vi "Measurement Logic.vi"() -> ()   [LabVIEW 2021, in "Crosstalk_PMIC.lvlib"]
uses:
  Crosstalk_PMIC.lvlib
  Measurement Configuration.ctl
  Measurement Results.ctl
  <vilib>/MeasurementLink/MeasurementLink Measurement Server/Measure Call Context/Measure Call Context.lvclass
  <instrlib>/niDCPower/nidcpower.llb/niDCPower Sense.ctl
  <instrlib>/niDCPower/nidcpower.llb/niDCPower Source Mode.ctl
  <instrlib>/niDCPower/nidcpower.llb/niDCPower Wait For Event - Event.ctl
  <instrlib>/niDCPower/nidcpower.llb/niDCPower Measurement Type.ctl
  <instrlib>/niScope/Controls/niScope vertical coupling.ctl
  <instrlib>/niScope/Controls/niScope trigger slope.ctl
  <instrlib>/niScope/Controls/niScope trigger coupling.ctl
  <instrlib>/niScope/Controls/niScope trigger source.ctl
  <instrlib>/niDCPower/nidcpower.llb/niDCPower Get Channel Name From String.vi
  <instrlib>/niScope/Configure/Trigger/niScope Configure Trigger Edge.vi
  <instrlib>/niScope/Acquire/Fetch/niScope Multi Fetch WDT.vi
  <vilib>/MeasurementLink/MeasurementLink Measurement Server/Measure Call Context/Accessor/Is Canceled.vi
panel:
  out "CrosstalkGraph":waveform(dbl)[](graph) caption="Ripple"
  out "measure call context out":refnum<class "Measure Call Context.lvclass">
  in  "measure call context in":refnum<class "Measure Call Context.lvclass">
  out "measurement results":T1
  in  "measurement configuration":T2={"Mode of operation"=enum."Perform measurement", "DUT setup time"=1.0, "Aperture time"=0.005, "Source resource name"="", "Source voltage level"=6.0, "Source current limit"=25.0, "Load resource name"="", "Load voltage limit range"=6.0, "Load current level"=0.005, "Scope resource names"=[], "Scope channel names"=[], "Scope sample rate"=10000.0, "Scope acquisition time"=3.0, "Scope probe attenuation"=1.0, "ExportData"=FALSE}
  out "error out":errorcluster
  in  "error in":errorcluster
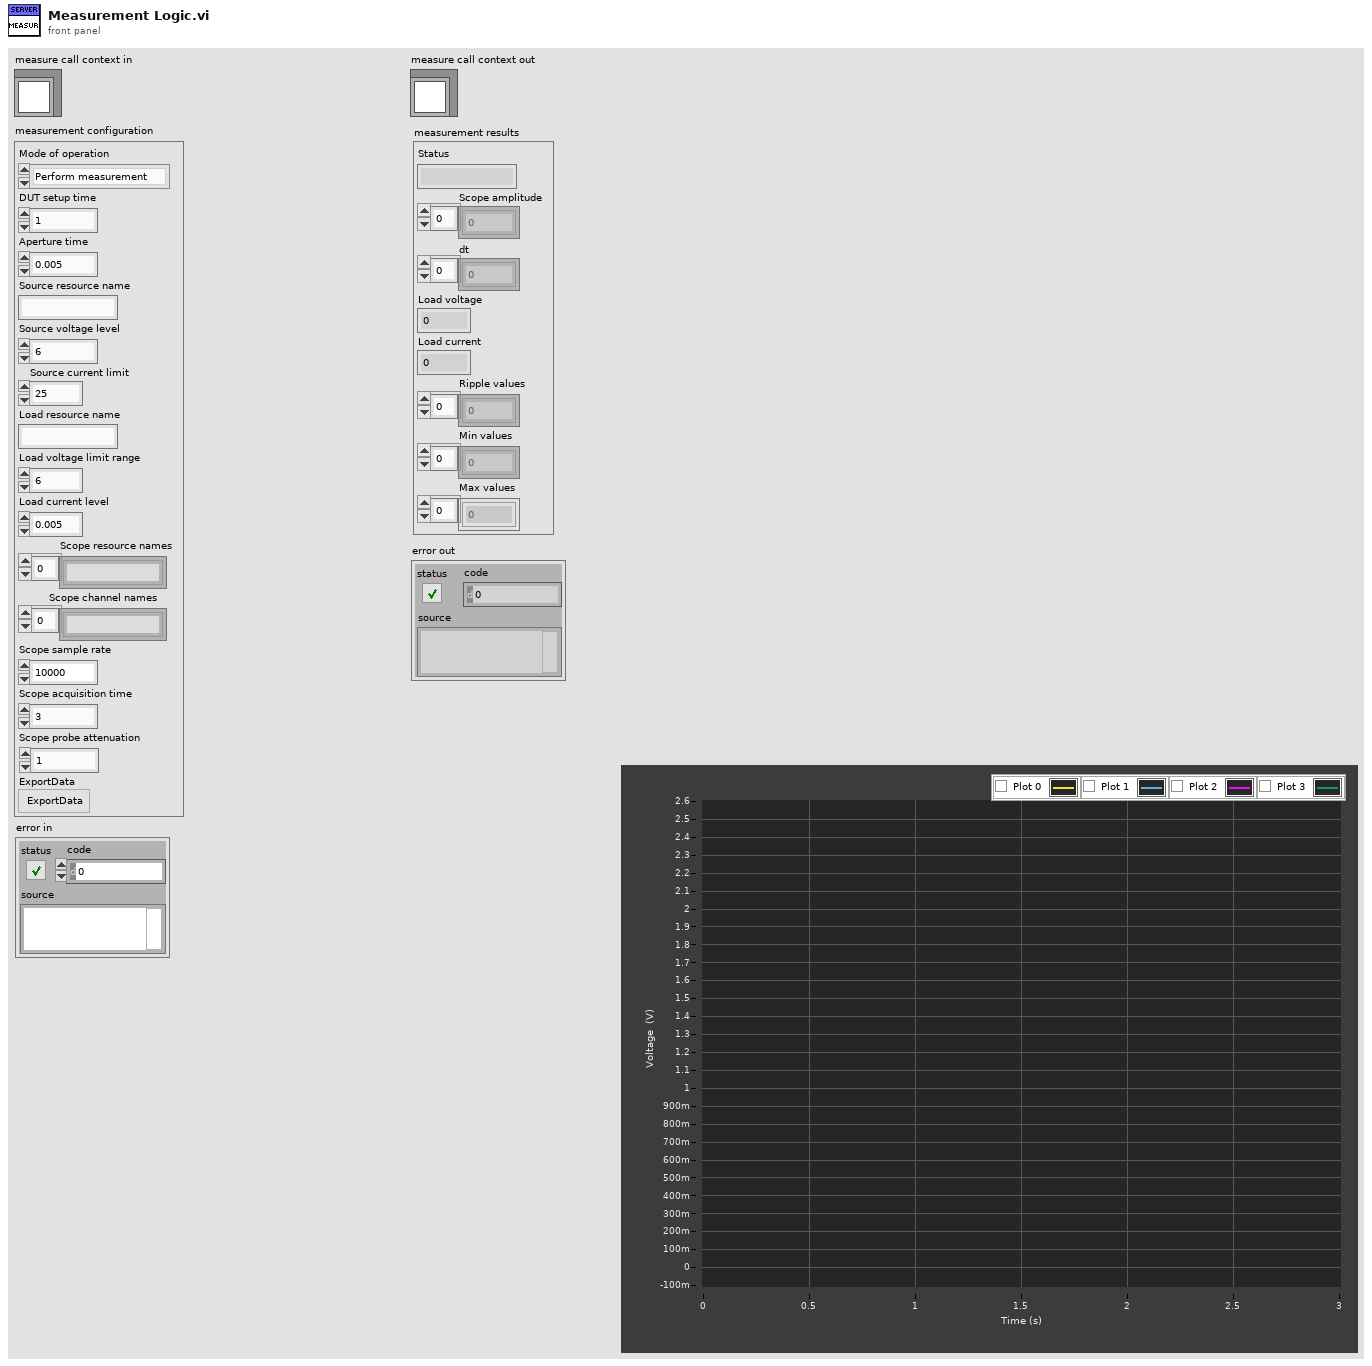
[diagram p1: front panel]
types:
  T1 = typedef "Crosstalk_PMIC.lvlib/Measurement Results.ctl" = cluster{"Status":string, "Scope amplitude":dbl[], "dt":dbl[], "Load voltage":dbl, "Load current":dbl, "Ripple values":dbl[], "Min values":dbl[], "Max values":dbl[]}
  T2 = typedef "Crosstalk_PMIC.lvlib/Measurement Configuration.ctl" = cluster{"Mode of operation":enum32{"Power on the DUT", "Perform measurement", "Power off the DUT"}, "DUT setup time":dbl, "Aperture time":dbl, "Source resource name":string, "Source voltage level":dbl, "Source current limit":dbl, "Load resource name":string, "Load voltage limit range":dbl, "Load current level":dbl, "Scope resource names":string[], "Scope channel names":string[], "Scope sample rate":dbl, "Scope acquisition time":dbl, "Scope probe attenuation":dbl, "ExportData":bool}
  T3 = cluster{"Source out":refnum<k15>, "Source channel name":string, "Load out":refnum<k15>, "Load channel name":string, "Scopes out":refnum<k15>[], "Scope channel names":string[], "Measurement Results":T1}
  T4 = enum32{"Power on the DUT", "Perform measurement", "Power off the DUT"}
  T5 = typedef "niScope trigger source.ctl" = string
  T6 = enum16{"open", "replace", "create", "open or create", "replace or create", "replace or create with confirmation"}
  T7 = typedef "niDCPower Wait For Event - Event.ctl" = i32
  T8 = typedef "niDCPower Source Mode.ctl" = i32
  T9 = typedef "niDCPower Sense.ctl" = i32
  T10 = typedef "niDCPower Measurement Type.ctl" = i32
  T11 = typedef "niScope vertical coupling.ctl" = i32
  T12 = typedef "niScope trigger coupling.ctl" = u16
  T13 = typedef "niScope trigger slope.ctl" = i32
  T14 = typedef "imagedata.ctl" = cluster{"image type":i32, "image depth":i32, "image":u8[], "mask":u8[], "colors":u32[], "Rectangle":cluster{"left":i16, "top":i16, "right":i16, "bottom":i16}}
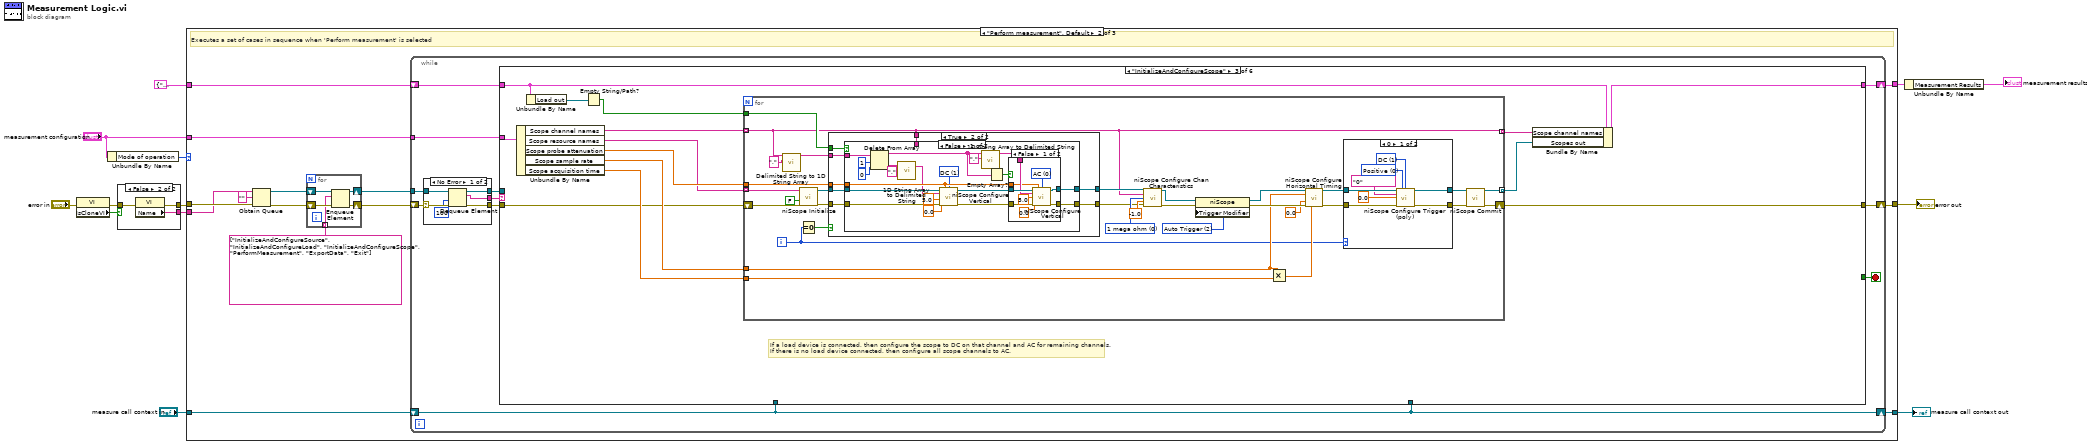
[diagram p0: block diagram]
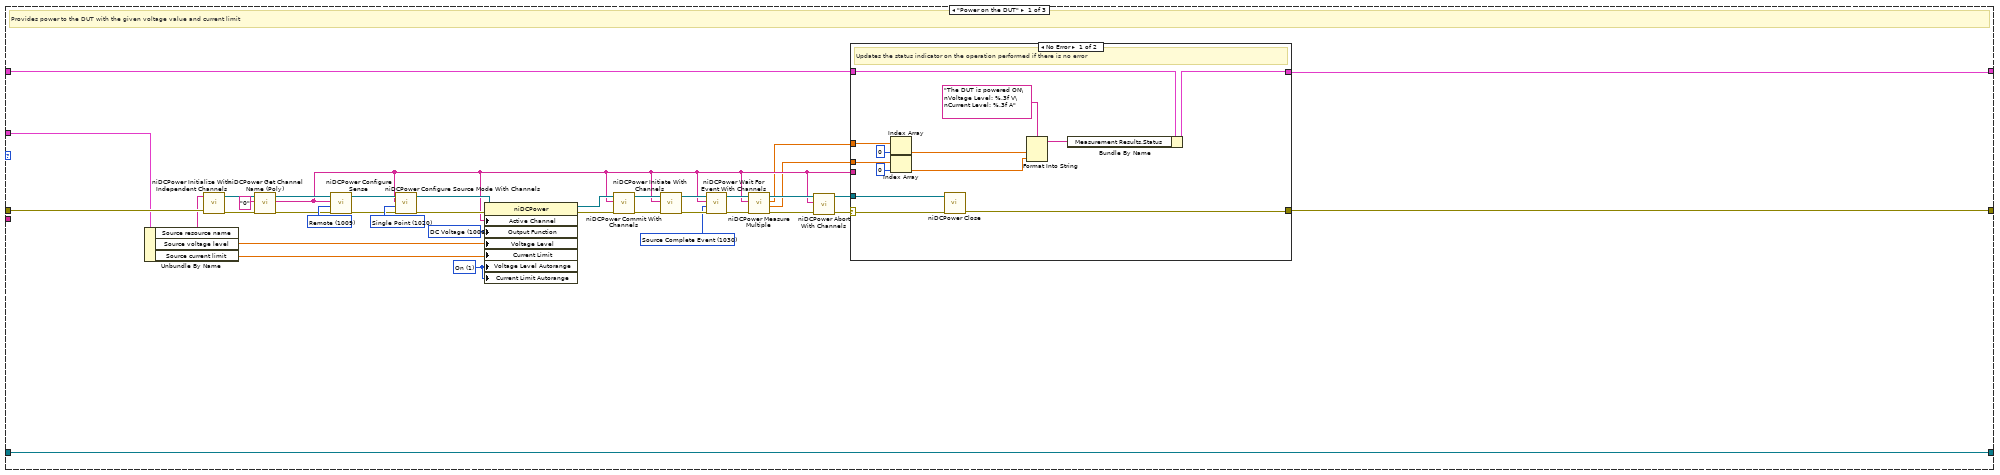
[diagram p2: hidden frame]
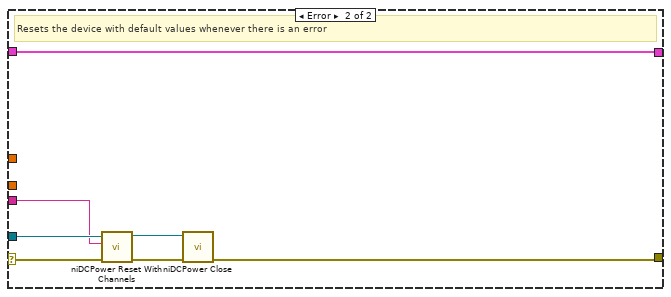
[diagram p3: hidden frame]
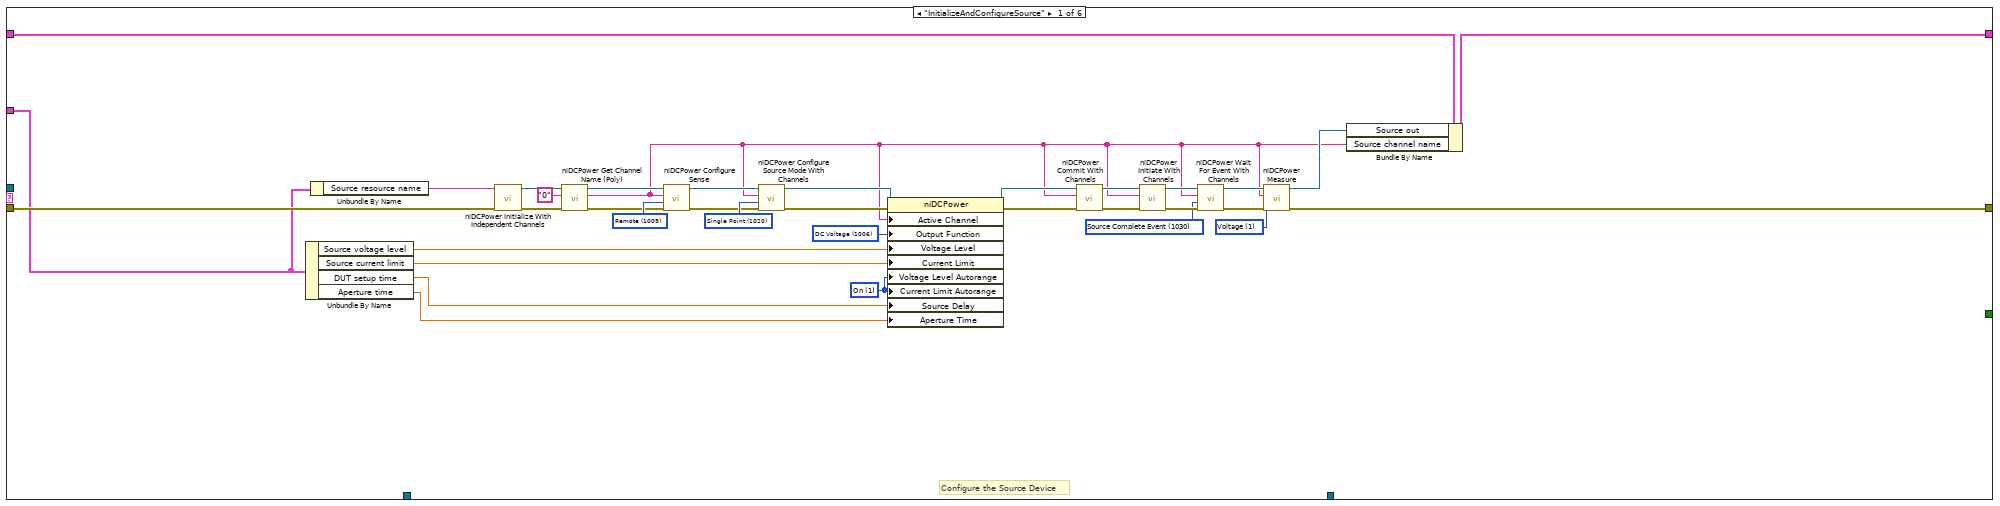
[diagram p4: hidden frame]
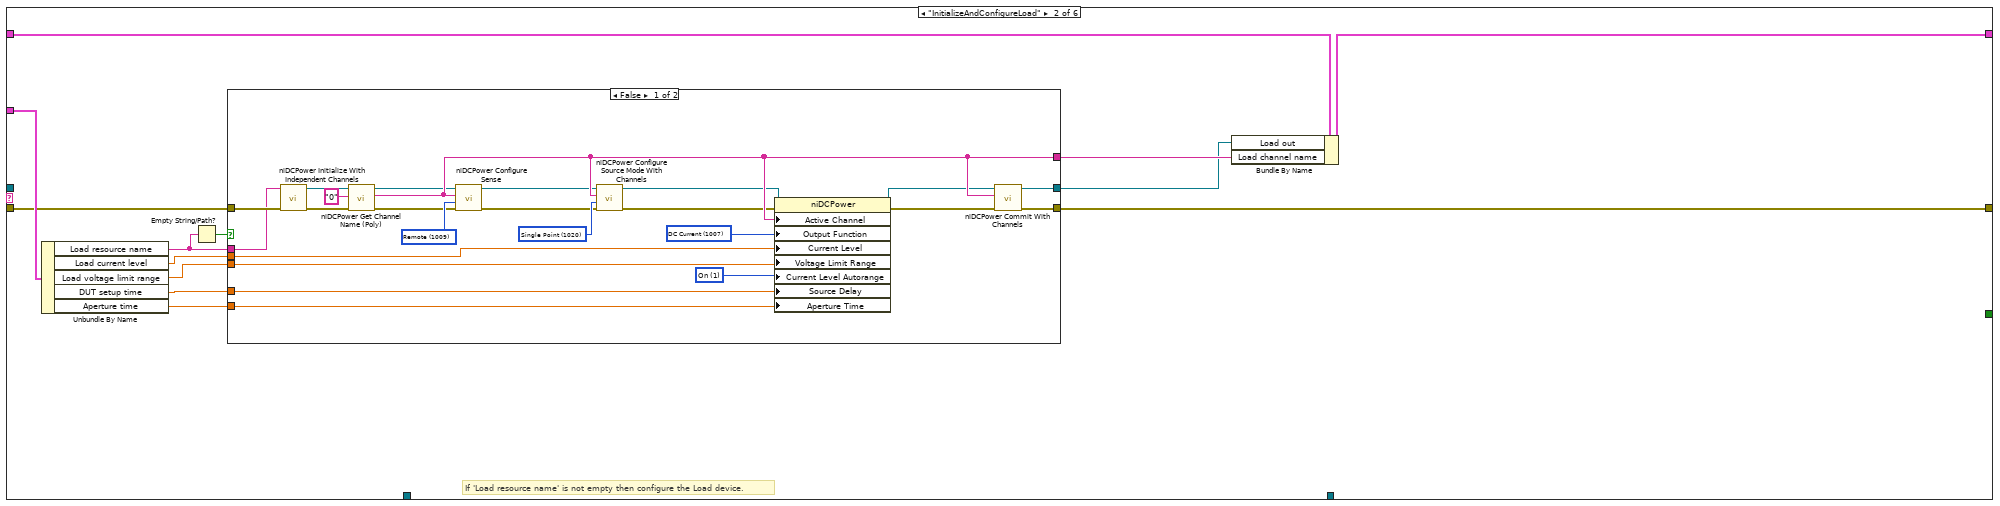
[diagram p5: hidden frame]
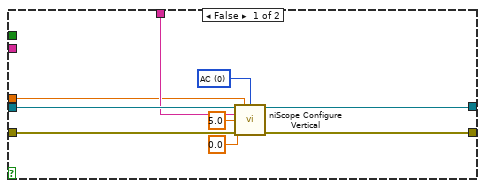
[diagram p7: hidden frame]
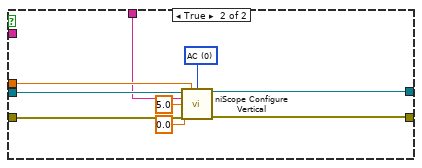
[diagram p9: hidden frame]
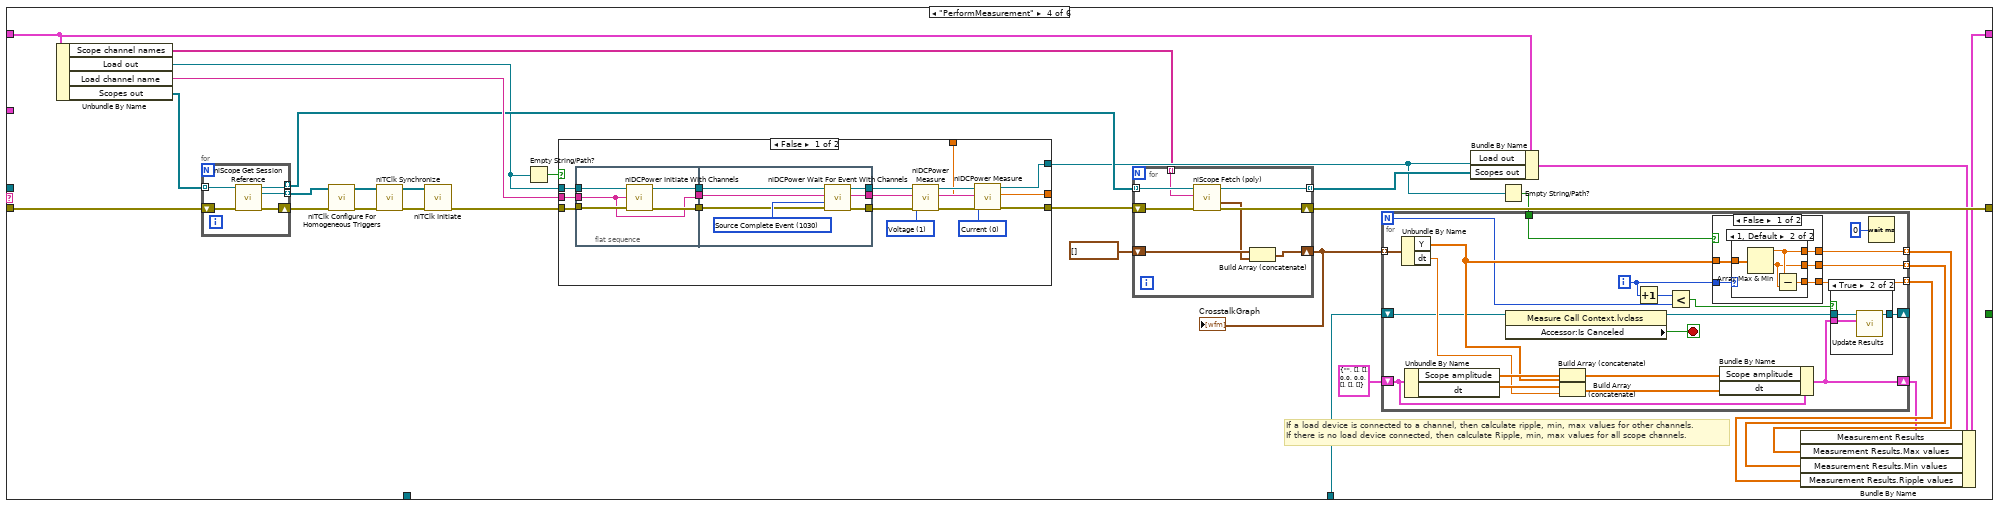
[diagram p11: hidden frame]
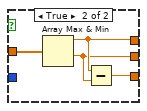
[diagram p15: hidden frame]
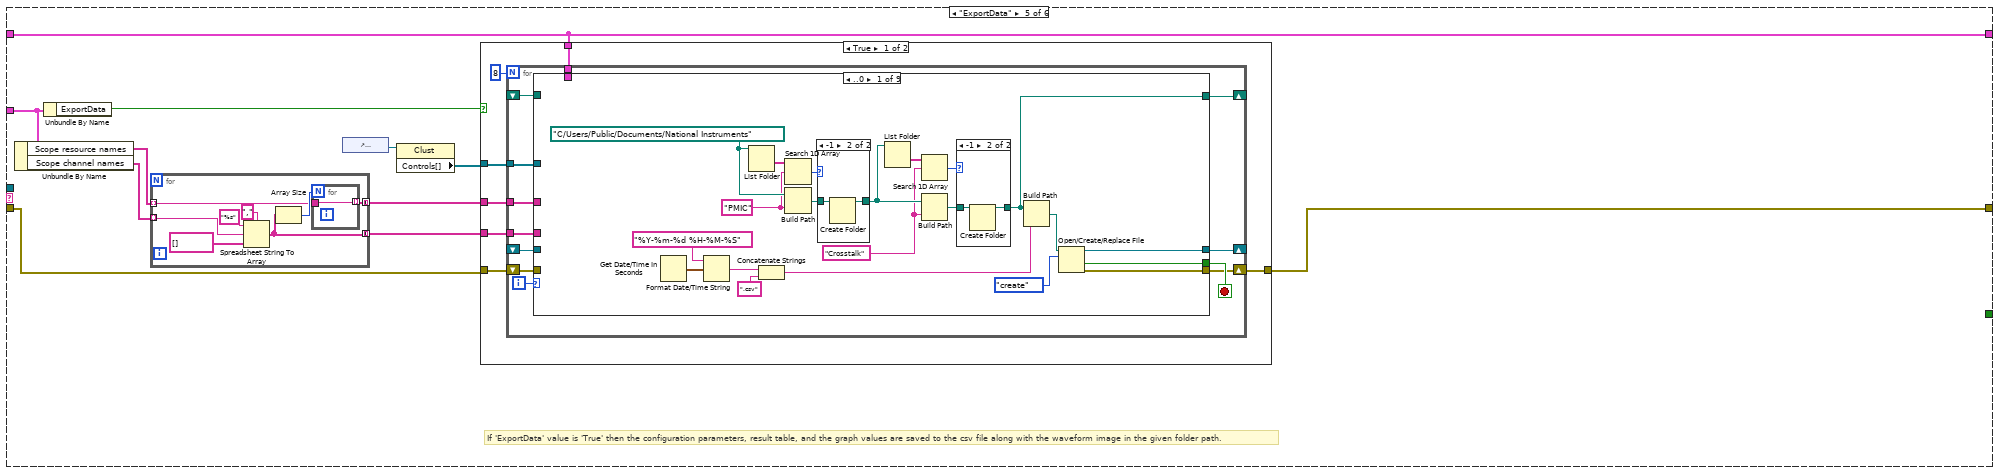
[diagram p16: hidden frame]
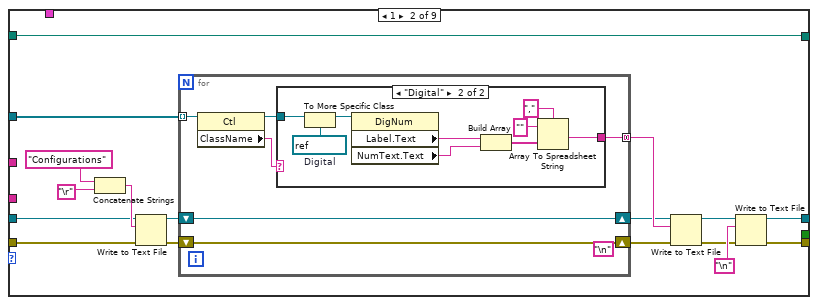
[diagram p19: hidden frame]
diagram:
  n1 = property class="VI"(error in="error in") -> (error out=w12:errorcluster, "IsCloneVI"=w13:bool)  [unwired: 1 in, 1 out]
  n2 = Unbundle By Name("measurement configuration") -> ("Mode of operation"=w7:T4)
  n3 = case shown="False" w13 {
    tunnel: [w16 w19] -> w10
    tunnel: [w15 w18] -> w9
    tunnel: w12 -> [w14 w17]
    frame True {
      n4 = property class="VI"(error in=w14) -> (error out=w16:errorcluster, "Clone Name"=w15:string)  [unwired: 1 in, 1 out]
    }
    frame False {
      n5 = property class="VI"(error in=w17) -> (error out=w19:errorcluster, "Name"=w18:string)  [unwired: 1 in, 1 out]
    }
  }
  n6 = case shown="\"Perform measurement\", Default" w7 {
    tunnel: [w21 w77 w717] -> w4
    tunnel: w10 -> [w37 w87 w716]
    tunnel: w9 -> [_ w86 _]
    tunnel: "measurement configuration" -> [w30 w83 w706]
    tunnel: [w22 w78 w703] -> w2
    tunnel: T3 {"Source out"="", "Source channel name"="", "Load out"="", "Load channel name"="", "Scopes out"=[], "Scope channel names"=[], "Measurement Results"={"Status"="", "Scope amplitude"=[], "dt"=[], "Load voltage"=0.0, "Load current"=0.0, "Ripple values"=[], "Min values"=[], "Max values"=[]}} -> [w23 w82 w704]
    tunnel: "measure call context in" -> [w20 w80 w705]
    tunnel: [w20 w79 w705] -> w5
    frame "Power on the DUT" {
      w40 = 1 items=["Off", "On"] ("Source:DC Voltage:Voltage Level Autorange")
      w41 = T7 1030 items=["Source Complete Event"=1030, "Measure Complete Event"=1031, "Sequence Iteration Complete Event"=1032, "Sequence Engine Done Event"=1033, "Pulse Complete Event"=1051, "Ready For Pulse Trigger Event"=1052] ("event")
      w52 = T8 1020 items=["Single Point"=1020, "Sequence"=1021] ("source mode")
      w47 = 1006 items=["DC Voltage"=1006, "DC Current"=1007, "Pulse Voltage"=1049, "Pulse Current"=1050] ("Source:Output Function")
      w42 = T9 1009 items=["Local"=1008, "Remote"=1009] ("sense")
      # "Provides power to the DUT with the given voltage value and current limit"
      n7 = Unbundle By Name(w30) -> ("Source resource name"=w34:string, "Source voltage level"=w29:dbl, "Source current limit"=w35:dbl)
      n8 = call <instrlib>:"niDCPower Initialize With Independent Channels.vi"("error in (no error)"=w37, "resource name"=w34) -> ("error out"=w39:errorcluster, "instrument handle out"=w43:refnum<k15>)  [unwired: 8 in]
      n9 = call-poly <instrlib>:"niDCPower Get Channel Name (Poly).vi"("index"="0", "instrument handle"=w43) -> ("name"=w26:string, "instrument handle out"=w38:refnum<k15>)  [unwired: 7 in, 1 out]
      n10 = call <instrlib>:"niDCPower Configure Sense.vi"("error in (no error)"=w39, "sense"=w42, "channel name"=w26, "instrument handle"=w38) -> ("error out"=w50:errorcluster, "instrument handle out"=w48:refnum<k15>)  [unwired: 6 in]
      n11 = call <instrlib>:"niDCPower Configure Source Mode With Channels.vi"("error in (no error)"=w50, "source mode"=w52, "channel name"=w26, "instrument handle"=w48) -> ("error out"=w51:errorcluster, "instrument handle out"=w49:refnum<k15>)  [unwired: 6 in]
      n12 = property class="niDCPower"(reference=w49, error in=w51, "Active Channel"=w26, "Output Function"=w47, "Voltage Level"=w29, "Current Limit"=w35, "Voltage Level Autorange"=w40, "Current Limit Autorange"=w40) -> (reference out=w53:refnum<k15>, error out=w54:errorcluster)
      n13 = call <instrlib>:"niDCPower Commit With Channels.vi"("error in (no error)"=w54, "channel name"=w26, "instrument handle"=w53) -> ("error out"=w56:errorcluster, "instrument handle out"=w55:refnum<k15>)  [unwired: 7 in]
      n14 = call <instrlib>:"niDCPower Initiate With Channels.vi"("error in (no error)"=w56, "channel name"=w26, "instrument handle"=w55) -> ("error out"=w44:errorcluster, "instrument handle out"=w45:refnum<k15>)  [unwired: 7 in]
      n15 = call <instrlib>:"niDCPower Wait For Event With Channels.vi"("error in (no error)"=w44, "event"=w41, "channel name"=w26, "instrument handle"=w45) -> ("error out"=w32:errorcluster, "instrument handle out"=w46:refnum<k15>)  [unwired: 6 in]
      n16 = call <instrlib>:"niDCPower Measure Multiple.vi"("error in (no error)"=w32, "channel name"=w26, "instrument handle"=w46) -> ("error out"=w31:errorcluster, "current measurements"=w24:dbl[], "voltage measurements"=w25:dbl[], "instrument handle out"=w33:refnum<k15>)  [unwired: 5 in]
      n17 = call <instrlib>:"niDCPower Abort With Channels.vi"("error in (no error)"=w31, "channel name"=w26, "instrument handle"=w33) -> ("error out"=w28:errorcluster, "instrument handle out"=w27:refnum<k15>)  [unwired: 7 in]
      n18 = case shown="No Error" w28 {
        selector: w28 -> [w69 w74]
        tunnel: [w68 w73] -> w21
        tunnel: [w67 w70] -> w22
        tunnel: w27 -> [w63 w72]
        tunnel: w26 -> [_ w71]
        tunnel: w25 -> [w62 _]
        tunnel: w24 -> [w61 _]
        tunnel: w23 -> [w60 w70]
        frame No Error {
          # "Updates the status indicator on the operation performed if there is no error"
          n19 = Index Array(array=w62, index=0) -> (element=w59:dbl)
          n20 = Index Array(array=w61, index=0) -> (element=w58:dbl)
          n21 = call <instrlib>:"niDCPower Close.vi"("error in (no error)"=w69, "instrument handle"=w63) -> ("error out"=w68:errorcluster)  [unwired: 9 out]
          n22 = Format Into String(format string="The DUT is powered ON\nVoltage Level: %.3f V\nCurrent Level: %.3f A" ("message"), w59, w58) -> (resulting string=w57:string)  [unwired: 2 in, 1 out]
          n23 = Bundle By Name(cluster=w60, "Measurement Results.Status"=w57) -> (w67:T3)
        }
        frame Error {
          # "Resets the device with default values whenever there is an error"
          n24 = call <instrlib>:"niDCPower Reset With Channels.vi"("error in (no error)"=w74, "channel name"=w71, "instrument handle"=w72) -> ("error out"=w76:errorcluster, "instrument handle out"=w75:refnum<k15>)  [unwired: 7 in]
          n25 = call <instrlib>:"niDCPower Close.vi"("error in (no error)"=w76, "instrument handle"=w75) -> ("error out"=w73:errorcluster)  [unwired: 9 out]
        }
      }
    }
    frame "Perform measurement", Default {
      # "Executes a set of cases in sequence when 'Perform measurement' is selected"
      n26 = Obtain Queue(name (unnamed)=w86, element data type="", error in (no error)=w87) -> (queue out=w89:refnum<queue>, error out=w90:errorcluster)  [unwired: 2 in, 1 out]
      n27 = for {
        shift-right: [w688] -> w84
        shift-left: w89 -> [w690]
        shift-right: [w687] -> w81
        shift-left: w90 -> [w689]
        tunnel: string[] ["InitializeAndConfigureSource", "InitializeAndConfigureLoad", "InitializeAndConfigureScope", "PerformMeasurement", "ExportData", "Exit"] ("Step sequence") -> [w686] mode=indexing
        n28 = Enqueue Element(queue=w690, element=w686, error in (no error)=w689) -> (queue out=w688:refnum<queue>, error out=w687:errorcluster)  [unwired: 1 in, 1 out]
      }
      n29 = while {
        tunnel: w84 -> [w101]
        tunnel: w83 -> [w98]
        shift-right: [w95] -> w78
        shift-left: w82 -> [w96]
        shift-right: [w94] -> w77
        shift-left: w81 -> [w100]
        shift-right: [w91] -> w79
        shift-left: w80 -> [w91]
        stop <- w93 stop-if-true
        n30 = case shown="No Error" w100 {
          selector: w100 -> [w680 w684]
          tunnel: w101 -> [w682 w683]
          tunnel: [w681 "Exit" ("t")] -> w92
          tunnel: [w679 w684] -> w97
          tunnel: [w677 w683] -> w99
          frame No Error {
            n31 = Dequeue Element(queue=w682, timeout in ms (-1)=100, error in (no error)=w680) -> (queue out=w677:refnum<queue>, element=w681:string, error out=w679:errorcluster)  [unwired: 1 out]
          }
          frame Error {
          }
        }
        n32 = case shown="\"InitializeAndConfigureScope\"" w92 {
          tunnel: w99 -> [_ _ _ _ _ w619]
          tunnel: w98 -> [w111 w149 w188 _ w405 _]
          tunnel: w97 -> [w113 w148 w182 w305 w407 w624]
          tunnel: w96 -> [w133 w144 w177 w315 w399 w622]
          tunnel: [w134 w146 w183 w309 w399 w620] -> w95
          tunnel: [w136 w147 w181 w313 w406 w621] -> w94
          tunnel: w91 -> [_ _ _ _ _ _]
          tunnel: [_ _ _ _ _ TRUE] -> w93
          tunnel: w91 -> [_ _ _ w288 _ _]
          frame "InitializeAndConfigureSource" {
            w102 = T10 1 items=["Current", "Voltage"] ("measurement type")
            w115 = 1 items=["Off", "On"] ("Source:DC Voltage:Voltage Level Autorange")
            w116 = T7 1030 items=["Source Complete Event"=1030, "Measure Complete Event"=1031, "Sequence Iteration Complete Event"=1032, "Sequence Engine Done Event"=1033, "Pulse Complete Event"=1051, "Ready For Pulse Trigger Event"=1052] ("event")
            w128 = T8 1020 items=["Single Point"=1020, "Sequence"=1021] ("source mode")
            w123 = 1006 items=["DC Voltage"=1006, "DC Current"=1007, "Pulse Voltage"=1049, "Pulse Current"=1050] ("Source:Output Function")
            w117 = T9 1009 items=["Local"=1008, "Remote"=1009] ("sense")
            # "Configure the Source Device"
            n33 = Unbundle By Name(w111) -> ("Source voltage level"=w104:dbl, "Source current limit"=w112:dbl, "DUT setup time"=w114:dbl, "Aperture time"=w103:dbl)
            n34 = Unbundle By Name(w111) -> ("Source resource name"=w110:string)
            n35 = call <instrlib>:"niDCPower Initialize With Independent Channels.vi"("error in (no error)"=w113, "resource name"=w110) -> ("error out"=w106:errorcluster, "instrument handle out"=w118:refnum<k15>)  [unwired: 8 in]
            n36 = call-poly <instrlib>:"niDCPower Get Channel Name (Poly).vi"("error in (no error)"=w106, "index"="0", "instrument handle"=w118) -> ("error out"=w105:errorcluster, "name"=w107:string, "instrument handle out"=w109:refnum<k15>)  [unwired: 6 in]
            n37 = call <instrlib>:"niDCPower Configure Sense.vi"("error in (no error)"=w105, "sense"=w117, "channel name"=w107, "instrument handle"=w109) -> ("error out"=w126:errorcluster, "instrument handle out"=w124:refnum<k15>)  [unwired: 6 in]
            n38 = call <instrlib>:"niDCPower Configure Source Mode With Channels.vi"("error in (no error)"=w126, "source mode"=w128, "channel name"=w107, "instrument handle"=w124) -> ("error out"=w127:errorcluster, "instrument handle out"=w125:refnum<k15>)  [unwired: 6 in]
            n39 = property class="niDCPower"(reference=w125, error in=w127, "Active Channel"=w107, "Output Function"=w123, "Voltage Level"=w104, "Current Limit"=w112, "Voltage Level Autorange"=w115, "Current Limit Autorange"=w115, "Source Delay"=w114, "Aperture Time"=w103) -> (reference out=w129:refnum<k15>, error out=w130:errorcluster)
            n40 = call <instrlib>:"niDCPower Commit With Channels.vi"("error in (no error)"=w130, "channel name"=w107, "instrument handle"=w129) -> ("error out"=w132:errorcluster, "instrument handle out"=w131:refnum<k15>)  [unwired: 7 in]
            n41 = call <instrlib>:"niDCPower Initiate With Channels.vi"("error in (no error)"=w132, "channel name"=w107, "instrument handle"=w131) -> ("error out"=w119:errorcluster, "instrument handle out"=w120:refnum<k15>)  [unwired: 7 in]
            n42 = call <instrlib>:"niDCPower Wait For Event With Channels.vi"("error in (no error)"=w119, "event"=w116, "channel name"=w107, "instrument handle"=w120) -> ("error out"=w122:errorcluster, "instrument handle out"=w121:refnum<k15>)  [unwired: 6 in]
            n43 = call <instrlib>:"niDCPower Measure.vi"("error in (no error)"=w122, "measurement type"=w102, "channel name"=w107, "instrument handle"=w121) -> ("error out"=w136:errorcluster, "instrument handle out"=w135:refnum<k15>)  [unwired: 5 in, 1 out]
            n44 = Bundle By Name(cluster=w133, "Source out"=w135, "Source channel name"=w107) -> (w134:T3)
          }
          frame "InitializeAndConfigureLoad" {
            # "If 'Load resource name' is not empty then configure the Load device."
            n45 = Unbundle By Name(w149) -> ("Load resource name"=w138:string, "Load current level"=w140:dbl, "Load voltage limit range"=w141:dbl, "DUT setup time"=w145:dbl, "Aperture time"=w139:dbl)
            n46 = Empty String/Path?(string/path=w138) -> (empty?=w137:bool)
            n47 = case shown="False" w137 {
              tunnel: w148 -> [w173 w174]
              tunnel: [w172 w174] -> w147
              tunnel: w145 -> [w171 _]
              tunnel: [w170 _] -> w143
              tunnel: [w169 _] -> w142
              tunnel: w141 -> [w168 _]
              tunnel: w140 -> [w167 _]
              tunnel: w139 -> [w166 _]
              tunnel: w138 -> [w150 _]
              frame False {
                w163 = T8 1020 items=["Single Point"=1020, "Sequence"=1021] ("source mode")
                w155 = 1 items=["Off", "On"] ("Source:DC Current:Current Level Autorange")
                w157 = 1007 items=["DC Voltage"=1006, "DC Current"=1007, "Pulse Voltage"=1049, "Pulse Current"=1050] ("Source:Output Function")
                w156 = T9 1009 items=["Local"=1008, "Remote"=1009] ("sense")
                n48 = call <instrlib>:"niDCPower Initialize With Independent Channels.vi"("error in (no error)"=w173, "resource name"=w150) -> ("error out"=w152:errorcluster, "instrument handle out"=w158:refnum<k15>)  [unwired: 8 in]
                n49 = call-poly <instrlib>:"niDCPower Get Channel Name (Poly).vi"("error in (no error)"=w152, "index"="0", "instrument handle"=w158) -> ("error out"=w151:errorcluster, "name"=w170:string, "instrument handle out"=w154:refnum<k15>)  [unwired: 6 in]
                n50 = call <instrlib>:"niDCPower Configure Sense.vi"("error in (no error)"=w151, "sense"=w156, "channel name"=w170, "instrument handle"=w154) -> ("error out"=w160:errorcluster, "instrument handle out"=w159:refnum<k15>)  [unwired: 6 in]
                n51 = call <instrlib>:"niDCPower Configure Source Mode With Channels.vi"("error in (no error)"=w160, "source mode"=w163, "channel name"=w170, "instrument handle"=w159) -> ("error out"=w162:errorcluster, "instrument handle out"=w161:refnum<k15>)  [unwired: 6 in]
                n52 = property class="niDCPower"(reference=w161, error in=w162, "Active Channel"=w170, "Output Function"=w157, "Current Level"=w167, "Voltage Limit Range"=w168, "Current Level Autorange"=w155, "Source Delay"=w171, "Aperture Time"=w166) -> (reference out=w164:refnum<k15>, error out=w165:errorcluster)
                n53 = call <instrlib>:"niDCPower Commit With Channels.vi"("error in (no error)"=w165, "channel name"=w170, "instrument handle"=w164) -> ("error out"=w172:errorcluster, "instrument handle out"=w169:refnum<k15>)  [unwired: 7 in]
              }
              frame True {
              }
            }
            n54 = Bundle By Name(cluster=w144, "Load out"=w142, "Load channel name"=w143) -> (w146:T3)
          }
          frame "InitializeAndConfigureScope" {
            # "If a load device is connected, then configure the scope to DC on that channel and AC for remaining channels.\nIf there is no load device connected, then configure all scope channels to AC."
            n55 = Unbundle By Name(w188) -> ("Scope channel names"=w178:string[], "Scope resource names"=w179:string[], "Scope probe attenuation"=w187:dbl, "Scope sample rate"=w186:dbl, "Scope acquisition time"=w185:dbl)
            n56 = Unbundle By Name(w177) -> ("Load out"=w176:refnum<k15>)
            n57 = Empty String/Path?(string/path=w176) -> (empty?=w175:bool)
            n58 = for {
              tunnel: w179 -> [w206] mode=indexing
              tunnel: w178 -> [w191] mode=indexing
              tunnel: [w204] -> w184 mode=indexing
              tunnel: w187 -> [w193]
              tunnel: w186 -> [w203]
              tunnel: w185 -> [w202]
              shift-right: [w200] -> w181
              shift-left: w182 -> [w201]
              tunnel: [w191] -> w180 mode=indexing
              tunnel: w175 -> [w192]
              i -> [w190]
              w214 = 2 items=["None"=1, "Auto Trigger"=2] ("Triggering:Trigger Modifier")
              w218 = u32 0 items=["1 mega ohm"=0, "50 ohms"=2] ("input impedance")
              n59 = call <vilib>:"Delimited String to 1D String Array.vi"("delimiter"=",", "delimited string"=w191) -> ("string array"=w198:string[])  [unwired: 9 in]
              n60 = call <instrlib>:"niScope Initialize.vi"("resource name"=w206, "reset device"=FALSE, "error in"=w201) -> ("instrument handle"=w196:refnum<k15>, "error out"=w195:errorcluster)  [unwired: 11 in]
              n61 = Equal To 0?(x=w190) -> (x = 0?=w189:bool)
              n62 = case shown="True" w189 {
                tunnel: w198 -> [_ w236]
                tunnel: [w227 w235] -> w197
                tunnel: w196 -> [w228 w234]
                tunnel: w195 -> [w226 w233]
                tunnel: [w225 w232] -> w194
                tunnel: w193 -> [w220 w231]
                tunnel: w192 -> [_ w230]
                tunnel: w191 -> [w224 w229]
                frame False {
                  w223 = T11 0 items=["AC", "DC", "Ground"] ("vertical coupling")
                  n63 = call <instrlib>:"niScope Configure Vertical.vi"("instrument handle"=w228, "probe attenuation"=w220, "vertical coupling"=w223, "channels"=w224, "vertical range"=5.0, "vertical offset"=0.0, "error in"=w226) -> ("instrument handle out"=w227:refnum<k15>, "error out"=w225:errorcluster)  [unwired: 7 in]
                }
                frame True {
                  n64 = case shown="False" w230 {
                    tunnel: w236 -> [w256 _]
                    tunnel: [w252 w275] -> w235
                    tunnel: w234 -> [w251 w276]
                    tunnel: w233 -> [w250 w274]
                    tunnel: [w249 w273] -> w232
                    tunnel: w231 -> [w247 w269]
                    tunnel: w229 -> [_ w268]
                    frame False {
                      w242 = T11 1 items=["AC", "DC", "Ground"] ("vertical coupling")
                      n65 = Delete From Array(array=w256, length=1, index=0) -> (deleted portion=w245:string[], array with subset deleted=w237:string[])
                      n66 = call <vilib>:"1D String Array to Delimited String.vi"("delimiter"=",", "string array"=w245) -> ("delimited string"=w246:string)  [unwired: 9 in]
                      n67 = call <instrlib>:"niScope Configure Vertical.vi"("instrument handle"=w251, "probe attenuation"=w247, "vertical coupling"=w242, "channels"=w246, "vertical range"=5.0, "vertical offset"=0.0, "error in"=w250) -> ("instrument handle out"=w253:refnum<k15>, "error out"=w248:errorcluster)  [unwired: 7 in]
                      n68 = call <vilib>:"1D String Array to Delimited String.vi"("delimiter"=",", "string array"=w237) -> ("delimited string"=w238:string)  [unwired: 9 in]
                      n69 = Empty Array?(array=w237) -> (empty?=w239:bool)
                      n70 = case shown="False" w239 {
                        tunnel: w253 -> [w265 w267]
                        tunnel: w238 -> [w264 _]
                        tunnel: [w263 w267] -> w252
                        tunnel: [w262 w266] -> w249
                        tunnel: w248 -> [w261 w266]
                        tunnel: w247 -> [w257 _]
                        frame False {
                          w259 = T11 0 items=["AC", "DC", "Ground"] ("vertical coupling")
                          n71 = call <instrlib>:"niScope Configure Vertical.vi"("instrument handle"=w265, "probe attenuation"=w257, "vertical coupling"=w259, "channels"=w264, "vertical range"=5.0, "vertical offset"=0.0, "error in"=w261) -> ("instrument handle out"=w263:refnum<k15>, "error out"=w262:errorcluster)  [unwired: 7 in]
                        }
                        frame True {
                        }
                      }
                    }
                    frame True {
                      w270 = T11 0 items=["AC", "DC", "Ground"] ("vertical coupling")
                      n72 = call <instrlib>:"niScope Configure Vertical.vi"("instrument handle"=w276, "probe attenuation"=w269, "vertical coupling"=w270, "channels"=w268, "vertical range"=5.0, "vertical offset"=0.0, "error in"=w274) -> ("instrument handle out"=w275:refnum<k15>, "error out"=w273:errorcluster)  [unwired: 7 in]
                    }
                  }
                }
              }
              n73 = call <instrlib>:"niScope Configure Chan Characteristics.vi"("instrument handle"=w197, "channels"=w191, "input impedance"=w218, "maximum input frequency"=-1.0, "error in"=w194) -> ("instrument handle out"=w216:refnum<k15>, "error out"=w215:errorcluster)  [unwired: 9 in]
              n74 = property class="niScope"(reference=w216, error in=w215, "Trigger Modifier"=w214) -> (reference out=w213:refnum<k15>, error out=w212:errorcluster)
              n75 = Multiply(x=w203, y=w202) -> (x*y=w207:dbl)
              n76 = call <instrlib>:"niScope Configure Horizontal Timing.vi"("instrument handle"=w213, "min sample rate"=w203, "reference position"=0.0, "error in"=w212, "min record length"=w207) -> ("instrument handle out"=w211:refnum<k15>, "error out"=w210:errorcluster)  [unwired: 9 in]
              n77 = case shown="0" w190 {
                tunnel: w211 -> [w283 w286]
                tunnel: w210 -> [w282 w285]
                tunnel: [w280 w285] -> w208
                tunnel: [w281 w286] -> w205
                frame 0 {
                  w284 = T12 1 items=["AC"=0, "DC"=1, "HF Reject"=3, "LF Reject"=4, "AC Plus HF Reject"=1001] ("trigger coupling")
                  w279 = T13 0 items=["Positive", "Negative"] ("trigger slope")
                  n78 = call-poly <instrlib>:"niScope Configure Trigger (poly).vi"("instrument handle"=w283, "trigger slope"=w279, "trigger coupling"=w284, "trigger source"=T5 "0", "trigger level"=0.0, "error in"=w282) -> ("instrument handle out"=w281:refnum<k15>, "error out"=w280:errorcluster)  [unwired: 8 in]
                }
                frame 1, Default {
                }
              }
              n79 = call <instrlib>:"niScope Commit.vi"("instrument handle"=w205, "error in"=w208) -> ("instrument handle out"=w204:refnum<k15>, "error out"=w200:errorcluster)  [unwired: 12 in]
            }
            n80 = Bundle By Name(cluster=w177, "Scope channel names"=w180, "Scopes out"=w184) -> (w183:T3)
          }
          frame "PerformMeasurement" {
            # "If a load device is connected to a channel, then calculate ripple, min, max values for other channels.\nIf there is no load device connected, then calculate Ripple, min, max values for all scope channels."
            n81 = Unbundle By Name(w315) -> ("Scope channel names"=w291:string[], "Load out"=w304:refnum<k15>, "Load channel name"=w316:string, "Scopes out"=w306:refnum<k15>[])
            n82 = for {
              tunnel: [w319] -> w298 mode=indexing
              shift-right: [w320] -> w297
              shift-left: w305 -> [w321]
              tunnel: [w318] -> w308 mode=indexing
              tunnel: w306 -> [w317] mode=indexing
              n83 = call <instrlib>:"niScope Get Session Reference.vi"("instrument handle"=w317, "error in"=w321) -> ("instrument handle out"=w318:refnum<k15>, "session reference"=w319:refnum<k20>, "error out"=w320:errorcluster)  [unwired: 11 in]
            }
            n84 = call <instrlib>:"niTClk Configure For Homogeneous Triggers.vi"("error in (no error)"=w297, "sessions"=w298) -> ("error out"=w299:errorcluster, "sessions out"=w300:refnum<k20>[])  [unwired: 8 in]
            n85 = call <instrlib>:"niTClk Synchronize.vi"("error in (no error)"=w299, "sessions"=w300) -> ("error out"=w301:errorcluster, "sessions out"=w302:refnum<k20>[])  [unwired: 8 in]
            n86 = call <instrlib>:"niTClk Initiate.vi"("error in (no error)"=w301, "sessions"=w302) -> ("error out"=w307:errorcluster)  [unwired: 8 in, 1 out]
            n87 = Empty String/Path?(string/path=w304) -> (empty?=w303:bool)
            n88 = case shown="False" w303 {
              tunnel: w316 -> [w335 _]
              tunnel: [w334 w351] -> w296
              tunnel: [w333 w350] -> w314
              tunnel: w307 -> [w332 w350]
              tunnel: w304 -> [w324 w351]
              tunnel: [w323 _] -> _
              tunnel: [w322 _] -> _
              frame False {
                w325 = T10 0 items=["Current", "Voltage"] ("measurement type")
                w327 = T10 1 items=["Current", "Voltage"] ("measurement type")
                n89 = flat-sequence {
                  tunnel: [w343] -> w338
                  tunnel: [w342] -> w337
                  tunnel: w332 -> [w341]
                  tunnel: w324 -> [w339]
                  tunnel: [w340] -> w336
                  tunnel: w335 -> [w340]
                  tunnel: w338 -> [w348]
                  tunnel: w337 -> [w345]
                  tunnel: [w346] -> w330
                  tunnel: [w347] -> w331
                  tunnel: w336 -> [w344]
                  tunnel: [w344] -> w326
                  frame #0 {
                    n90 = call <instrlib>:"niDCPower Initiate With Channels.vi"("error in (no error)"=w341, "channel name"=w340, "instrument handle"=w339) -> ("error out"=w343:errorcluster, "instrument handle out"=w342:refnum<k15>)  [unwired: 7 in]
                  }
                  frame #1 {
                    w349 = T7 1030 items=["Source Complete Event"=1030, "Measure Complete Event"=1031, "Sequence Iteration Complete Event"=1032, "Sequence Engine Done Event"=1033] ("event")
                    n91 = call <instrlib>:"niDCPower Wait For Event With Channels.vi"("error in (no error)"=w348, "event"=w349, "channel name"=w344, "instrument handle"=w345) -> ("error out"=w346:errorcluster, "instrument handle out"=w347:refnum<k15>)  [unwired: 6 in]
                  }
                }
                n92 = call <instrlib>:"niDCPower Measure.vi"("error in (no error)"=w330, "measurement type"=w327, "channel name"=w326, "instrument handle"=w331) -> ("error out"=w328:errorcluster, "measurement"=w323:dbl, "instrument handle out"=w329:refnum<k15>)  [unwired: 5 in]
                n93 = call <instrlib>:"niDCPower Measure.vi"("error in (no error)"=w328, "measurement type"=w325, "channel name"=w326, "instrument handle"=w329) -> ("error out"=w333:errorcluster, "measurement"=w322:dbl, "instrument handle out"=w334:refnum<k15>)  [unwired: 5 in]
              }
              frame True {
              }
            }
            n94 = for {
              shift-right: [w397] -> w313
              shift-left: w314 -> [w398]
              tunnel: w308 -> [w396] mode=indexing
              shift-right: [w394] -> w290
              shift-left: waveform(dbl)[] [] -> [w395]
              tunnel: [w393] -> w312 mode=indexing
              tunnel: w291 -> [w392] mode=indexing
              n95 = call-poly <instrlib>:"niScope Fetch (poly).vi"("error in"=w398, "channels"=w392, "instrument handle"=w396) -> ("error out"=w397:errorcluster, "wfm"=w391:waveform(dbl)[], "instrument handle out"=w393:refnum<k15>)  [unwired: 5 in, 1 out]
              n96 = Build Array (concatenate)(w395, w391) -> (w394:waveform(dbl)[])
            }
            "CrosstalkGraph" <- w290
            n97 = Bundle By Name(cluster=w315, "Load out"=w296, "Scopes out"=w312) -> (w310:T3)
            n98 = Empty String/Path?(string/path=w296) -> (empty?=w295:bool)
            n99 = for {
              N -> [w357]
              tunnel: w290 -> [w373] mode=indexing
              tunnel: [w372] -> w294 mode=indexing
              tunnel: [w371] -> w293 mode=indexing
              tunnel: w295 -> [w370]
              tunnel: [w369] -> w292 mode=indexing
              shift-right: [w355] -> w287
              shift-left: T1 {"Status"="", "Scope amplitude"=[], "dt"=[], "Load voltage"=0.0, "Load current"=0.0, "Ripple values"=[], "Min values"=[], "Max values"=[]} ("Measurement Results") -> [w364]
              shift-right: [w353] -> _
              shift-left: w288 -> [w361]
              i -> [w358]
              stop <- w360 stop-if-true
              n100 = Unbundle By Name(w373) -> ("Y"=w367:dbl[], "dt"=w365:dbl)
              n101 = Unbundle By Name(w364) -> ("Scope amplitude"=w368:dbl[], "dt"=w366:dbl[])
              n102 = property class="Measure Call Context.lvclass"(reference=w361) -> (reference out=w354:refnum<class "Measure Call Context.lvclass">, "Accessor:Is Canceled"=w360:bool)  [unwired: 1 in, 1 out]
              n103 = Build Array (concatenate)(w368, w367) -> (w363:dbl[])
              n104 = Build Array (concatenate)(w366, w365) -> (w362:dbl[])
              n105 = Increment(x=w358) -> (x+1=w359:i32)
              n106 = Less?(x=w359, y=w357) -> (x < y?=w356:bool)
              n107 = case shown="False" w370 {
                tunnel: w367 -> [w381 w390]
                tunnel: [w380 w388] -> w372
                tunnel: [w379 w387] -> w371
                tunnel: w358 -> [w382 _]
                tunnel: [w378 w389] -> w369
                frame False {
                  n108 = case shown="1, Default" w382 {
                    tunnel: w381 -> [_ w386]
                    tunnel: [_ w385] -> w380
                    tunnel: [_ w384] -> w379
                    tunnel: [_ w383] -> w378
                    frame 0 {
                    }
                    frame 1, Default {
                      n109 = Array Max & Min(array=w386) -> (max value=w385:dbl, min value=w384:dbl)  [unwired: 2 out]
                      n110 = Subtract(x=w385, y=w384) -> (x-y=w383:dbl)
                    }
                  }
                }
                frame True {
                  n111 = Array Max & Min(array=w390) -> (max value=w388:dbl, min value=w387:dbl)  [unwired: 2 out]
                  n112 = Subtract(x=w388, y=w387) -> (x-y=w389:dbl)
                }
              }
              n113 = Bundle By Name(cluster=w364, "Scope amplitude"=w363, "dt"=w362) -> (w355:T1)
              n114 = case shown="True" w356 {
                tunnel: [w374 w377] -> w353
                tunnel: w355 -> [_ w376]
                tunnel: w354 -> [w374 w375]
                frame False {
                }
                frame True {
                  n115 = call <vilib>:"Update Results.vi"("measurement results"=w376, "measure call context in"=w375) -> ("measure call context out"=w377:refnum<class "Measure Call Context.lvclass">)  [unwired: 8 in, 1 out]
                }
              }
              n116 = Wait (ms)(milliseconds to wait=u32 0) -> ()  [unwired: 1 out]
            }
            n117 = Bundle By Name(cluster=w310, "Measurement Results"=w287, "Measurement Results.Max values"=w294, "Measurement Results.Min values"=w293, "Measurement Results.Ripple values"=w292) -> (w309:T3)
          }
          frame "ExportData" {
            # "If 'ExportData' value is 'True' then the configuration parameters, result table, and the graph values are saved to the csv file along with the waveform image in the given folder path."
            n118 = Unbundle By Name(w405) -> ("Scope resource names"=w404:string[], "Scope channel names"=w403:string[])
            n119 = Unbundle By Name(w405) -> ("ExportData"=w408:bool)
            n120 = for {
              tunnel: [w414] -> w400 mode=concatenating
              tunnel: [w412] -> w401 mode=concatenating
              tunnel: w404 -> [w411] mode=indexing
              tunnel: w403 -> [w410] mode=indexing
              n121 = Spreadsheet String To Array(delimiter (Tab)=",", format string="%s", spreadsheet string=w410, array type (2D Dbl)=string[] []) -> (array=w414:string[])
              n122 = Array Size(array=w414) -> (size(s)=w413:i32)
              n123 = for {
                N: w413 -> [_]
                tunnel: w411 -> [w418]
                tunnel: [w418] -> w412 mode=indexing
              }
            }
            n124 = control-ref of="measurement configuration"() -> (w409:refnum<vi>)
            n125 = property class="Clust"(reference=w409) -> ("Controls[]"=w402:refnum<vi>[])  [unwired: 1 in, 2 out]
            n126 = case shown="True" w408 {
              tunnel: w402 -> [w424 _]
              tunnel: w407 -> [w423 w617]
              tunnel: [w422 w617] -> w406
              tunnel: w401 -> [w421 _]
              tunnel: w400 -> [w420 _]
              tunnel: w399 -> [w419 _]
              frame True {
                n127 = for {
                  N: 8 -> [_]
                  shift-right: [w435] -> _
                  shift-left: _ -> [w434]
                  shift-right: [w433] -> w422
                  shift-left: w423 -> [w432]
                  tunnel: w424 -> [w431]
                  tunnel: w421 -> [w430]
                  tunnel: w420 -> [w429]
                  tunnel: w419 -> [w428]
                  shift-right: [w427] -> _
                  shift-left: _ -> [w426]
                  i -> [w437]
                  stop <- w436 stop-if-true
                  n128 = case shown="..0" w437 {
                    tunnel: [w451 _ _ _ _ _ _ _ _] -> w436
                    tunnel: [w457 w466 w504 w524 w557 refnum<file> refnum ("refnum out") w602 w612 w616] -> w435
                    tunnel: w434 -> [_ w477 w513 w531 w558 w590 w602 w612 w616]
                    tunnel: [w450 w468 w503 w523 w556 w588 w603 w613 w615] -> w433
                    tunnel: w432 -> [_ w475 w512 w530 w559 w587 w603 w613 w615]
                    tunnel: w431 -> [_ w478 _ _ _ _ _ _ _]
                    tunnel: w430 -> [_ _ _ w521 _ _ _ _ _]
                    tunnel: w429 -> [_ _ _ w520 _ _ _ _ _]
                    tunnel: w428 -> [_ _ _ w519 _ _ _ _ _]
                    tunnel: [w438 w465 w497 w514 w548 w586 w591 w606 w614] -> w427
                    tunnel: w426 -> [_ w465 w497 w514 w548 w586 w591 w606 w614]
                    frame ..0 {
                      w446 = "Crosstalk" ("prompt")
                      w453 = "PMIC" ("prompt")
                      w456 = path "C:/Users/Public/Documents/National Instruments" ("base path")
                      n129 = Get Date/Time In Seconds() -> (seconds since 1Jan1904=w443:timestamp)
                      n130 = Format Date/Time String(time format string (%c)="%Y-%m-%d %H-%M-%S", seconds (now)=w443) -> (date/time string=w442:string)  [unwired: 1 in]
                      n131 = List Folder(path=w456) -> (folder names=w454:string[])  [unwired: 3 in, 3 out]
                      n132 = Concatenate Strings(w442, ".csv" ("string")) -> (w440:string)
                      n133 = Search 1D Array(1D array=w454, element=w453) -> (index of element=w452:i32)  [unwired: 1 in]
                      n134 = Build Path(base path=w456, name or relative path=w453) -> (appended path=w455:path)
                      n135 = case shown="-1" w452 {
                        tunnel: w455 -> [w462 w464]
                        tunnel: [w462 w463] -> w447
                        frame Default {
                        }
                        frame -1 {
                          n136 = Create Folder(path (use dialog)=w464) -> (created path=w463:path)  [unwired: 2 in, 2 out]
                        }
                      }
                      n137 = List Folder(path=w447) -> (folder names=w449:string[])  [unwired: 3 in, 3 out]
                      n138 = Search 1D Array(1D array=w449, element=w446) -> (index of element=w448:i32)  [unwired: 1 in]
                      n139 = Build Path(base path=w447, name or relative path=w446) -> (appended path=w445:path)
                      n140 = case shown="-1" w448 {
                        tunnel: w445 -> [w459 w461]
                        tunnel: [w459 w460] -> w438
                        frame Default {
                        }
                        frame -1 {
                          n141 = Create Folder(path (use dialog)=w461) -> (created path=w460:path)  [unwired: 2 in, 2 out]
                        }
                      }
                      n142 = Build Path(base path=w438, name or relative path=w440) -> (appended path=w439:path)
                      n143 = Open/Create/Replace File(file path (use dialog)=w439, operation (0:open)=T6."create") -> (refnum out=w457:refnum<file>, cancelled=w451:bool, error out=w450:errorcluster)  [unwired: 4 in]
                    }
                    frame 1 {
                      (unwired) "\n"
                      n144 = Concatenate Strings("Configurations" ("format string"), "\r") -> (w479:string)
                      n145 = Write to Text File(file (use dialog)=w477, text=w479, error in=w475) -> (refnum out=w474:refnum<file>, error out=w476:errorcluster)  [unwired: 1 in, 1 out]
                      n146 = for {
                        tunnel: w478 -> [w483] mode=indexing
                        shift-right: [w487] -> w472
                        shift-left: w474 -> [w487]
                        shift-right: [w486] -> w471
                        shift-left: w476 -> [w486]
                        tunnel: [w485] -> w473 mode=concatenating
                        n147 = property class="Ctl"(reference=w483) -> (reference out=w484:refnum<vi>, "ClassName"=w482:string)  [unwired: 1 in, 1 out]
                        n148 = case shown="\"Digital\"" w482 {
                          tunnel: [_ w491] -> w485
                          tunnel: w484 -> [_ w489]
                          frame Default {
                          }
                          frame "Digital" {
                            w488 = refnum<vi> refnum  # Digital
                            n149 = To More Specific Class(target class=w488, reference=w489) -> (specific class reference=w490:refnum<vi>)  [unwired: 1 in, 1 out]
                            n150 = property class="DigNum"(reference=w490) -> ("Label.Text"=w496:string, "NumText.Text"=w495:string)  [unwired: 1 in, 2 out]
                            n151 = Build Array(w496, w495) -> (w492:string[])
                            n152 = Array To Spreadsheet String(delimiter (Tab)=",", array=w492, 3:"" ("format string")) -> (spreadsheet string=w491:string)
                          }
                        }
                      }
                      n153 = Write to Text File(file (use dialog)=w472, text=w473, error in=w471) -> (refnum out=w467:refnum<file>, error out=w469:errorcluster)  [unwired: 1 in, 1 out]
                      n154 = Write to Text File(file (use dialog)=w467, text="\n", error in=w469) -> (refnum out=w466:refnum<file>, error out=w468:errorcluster)  [unwired: 1 in, 1 out]
                    }
                    frame 2 {
                      n155 = Concatenate Strings("Results" ("element"), "\r") -> (w499:string)
                      n156 = Write to Text File(file (use dialog)=w513, text=w499, error in=w512) -> (refnum out=w511:refnum<file>, error out=w507:errorcluster)  [unwired: 1 in, 1 out]
                      n157 = Array To Spreadsheet String(delimiter (Tab)=",", array=string[] ["Scope", "Channel", "Pk-Pk Ripple (V) ", "Minimum (V)", "Maximum (V)"], 3:"" ("format string")) -> (spreadsheet string=w508:string)
                      n158 = Write to Text File(file (use dialog)=w511, text=w508, error in=w507) -> (refnum out=w506:refnum<file>, error out=w505:errorcluster)  [unwired: 1 in, 1 out]
                      n159 = Write to Text File(file (use dialog)=w506, text="\n", error in=w505) -> (refnum out=w504:refnum<file>, error out=w503:errorcluster)  [unwired: 1 in, 1 out]
                    }
                    frame 3 {
                      n160 = Unbundle By Name(w519) -> ("Measurement Results.Ripple values"=w518:dbl[], "Measurement Results.Min values"=w517:dbl[], "Measurement Results.Max values"=w516:dbl[])
                      n161 = for {
                        tunnel: [w541] -> w515 mode=indexing
                        tunnel: w518 -> [w540] mode=indexing
                        tunnel: w517 -> [w539] mode=indexing
                        tunnel: w516 -> [w538] mode=indexing
                        tunnel: w520 -> [w534] mode=indexing
                        tunnel: w521 -> [w535] mode=indexing
                        n162 = Build Array(w540, w539, w538) -> (w537:dbl[])
                        n163 = Build Array(w535, w534) -> (w533:string[])
                        n164 = for {
                          tunnel: w533 -> [w544] mode=indexing
                          tunnel: [w543] -> w532 mode=indexing
                          n165 = Format Into String(format string="%s" ("initial string"), w544) -> (resulting string=w543:string)  [unwired: 2 in, 1 out]
                        }
                        n166 = for {
                          tunnel: w537 -> [w547] mode=indexing
                          tunnel: [w546] -> w536 mode=indexing
                          n167 = Format Into String(format string="%.6f" ("initial string"), w547) -> (resulting string=w546:string)  [unwired: 2 in, 1 out]
                        }
                        n168 = Build Array (concatenate)(w532, w536) -> (w541:string[])
                      }
                      n169 = Array To Spreadsheet String(delimiter (Tab)=",", array=w515, 3:"" ("format string")) -> (spreadsheet string=w527:string)
                      n170 = Write to Text File(file (use dialog)=w531, text=w527, error in=w530) -> (refnum out=w526:refnum<file>, error out=w525:errorcluster)  [unwired: 1 in, 1 out]
                      n171 = Write to Text File(file (use dialog)=w526, text="\n", error in=w525) -> (refnum out=w524:refnum<file>, error out=w523:errorcluster)  [unwired: 1 in, 1 out]
                    }
                    frame 4 {
                      n172 = Concatenate Strings("Crosstalk" ("string"), "\r") -> (w571:string)
                      n173 = property on="CrosstalkGraph" class="WFGraph (strict)"() -> ("Value"=w549:waveform(dbl)[])  [unwired: 2 in, 2 out]
                      n174 = Write to Text File(file (use dialog)=w558, text=w571, error in=w559) -> (refnum out=w568:refnum<file>, error out=w567:errorcluster)  [unwired: 1 in, 1 out]
                      n175 = Build Array("Time (s)", "Voltage (V)") -> (w570:string[])
                      n176 = Array To Spreadsheet String(delimiter (Tab)=",", array=w570, 3:"" ("format string")) -> (spreadsheet string=w566:string)
                      n177 = for {
                        tunnel: [w585] -> w555 mode=indexing
                        tunnel: [w584] -> w554 mode=indexing
                        tunnel: w549 -> [w583] mode=indexing
                        n178 = Unbundle By Name(w583) -> ("dt"=w584:dbl, "Y"=w585:dbl[])
                      }
                      n179 = Write to Text File(file (use dialog)=w568, text=w566, error in=w567) -> (refnum out=w565:refnum<file>, error out=w564:errorcluster)  [unwired: 1 in, 1 out]
                      n180 = for {
                        tunnel: [w575] -> w561 mode=concatenating
                        tunnel: w555 -> [w574] mode=indexing
                        tunnel: w554 -> [w573] mode=indexing
                        n181 = for {
                          tunnel: [w580] -> w575 mode=indexing
                          tunnel: w574 -> [w579] mode=indexing
                          tunnel: w573 -> [w577]
                          i -> [w578]
                          n182 = Multiply(x=w577, y=w578) -> (x*y=w576:dbl)
                          n183 = Format Into String(w576) -> (resulting string=w581:string)  [unwired: 3 in, 1 out]
                          n184 = Format Into String(w579) -> (resulting string=w582:string)  [unwired: 3 in, 1 out]
                          n185 = Build Array(w581, w582) -> (w580:string[])
                        }
                      }
                      n186 = Array To Spreadsheet String(delimiter (Tab)=",", array=w561, 3:"" ("format string")) -> (spreadsheet string=w560:string)
                      n187 = Write to Text File(file (use dialog)=w565, text=w560, error in=w564) -> (refnum out=w557:refnum<file>, error out=w556:errorcluster)  [unwired: 1 in, 1 out]
                    }
                    frame 5 {
                      n188 = Close File(refnum=w590, error in=w587) -> (error out=w588:errorcluster)  [unwired: 1 out]
                    }
                    frame 6 {
                      n189 = Get Date/Time In Seconds() -> (seconds since 1Jan1904=w596:timestamp)
                      n190 = Format Date/Time String(time format string (%c)="%Y-%m-%d %H-%M-%S", seconds (now)=w596) -> (date/time string=w595:string)  [unwired: 1 in]
                      n191 = Concatenate Strings(w595, ".bmp" ("string")) -> (w593:string)
                      n192 = Build Path(base path=w591, name or relative path=w593) -> (appended path=w592:path)
                      n193 = invoke on="CrosstalkGraph" class="WFGraph (strict)" method="Export Image"("FileType"=enum32{"BMP", "EPS", "EMF", "PICT"}."BMP" ("File Type"), "Target"=enum32{"File", "Clipboard"}."File", "Path"=w592, "HideGrid"=TRUE ("Hide Grid"), "Overwrite"=FALSE ("Always Overwrite")) -> ()  [unwired: 3 in, 8 out]
                    }
                    frame 7 {
                      n194 = Get Date/Time In Seconds() -> (seconds since 1Jan1904=w610:timestamp)
                      n195 = Format Date/Time String(time format string (%c)="%Y-%m-%d %H-%M-%S", seconds (now)=w610) -> (date/time string=w609:string)  [unwired: 1 in]
                      n196 = Concatenate Strings(w609, ".png" ("string")) -> (w607:string)
                      n197 = Build Path(base path=w606, name or relative path=w607) -> (appended path=w604:path)
                      n198 = invoke on="CrosstalkGraph" class="WFGraph (strict)" method="Get Image"() -> ("image data"=w605:T14)  [unwired: 6 in, 5 out]
                      n199 = call <vilib>:"Write PNG File.vi"("image data"=w605, "path to PNG file"=w604) -> ()  [unwired: 8 in, 2 out]
                    }
                    frame Default {
                    }
                  }
                }
              }
              frame False {
              }
            }
          }
          frame "Exit", Default {
            # "Aborts and closes all the opened sessions"
            n200 = Release Queue(queue=w619, error in (no error)=w624) -> (error out=w623:errorcluster)  [unwired: 1 in, 2 out]
            n201 = case shown="No Error" w623 {
              selector: w623 -> [w630 w658]
              tunnel: [w631 w669] -> w621
              tunnel: w622 -> [w632 w668]
              tunnel: [w639 w668] -> w620
              frame No Error {
                # "Updates the status indicator on the operation performed if there is no error"
                n202 = Unbundle By Name(w632) -> ("Source out"=w638:refnum<k15>, "Source channel name"=w634:string, "Load out"=w626:refnum<k15>, "Load channel name"=w637:string, "Scopes out"=w628:refnum<k15>[])
                n203 = for {
                  shift-right: [w648] -> w629
                  shift-left: w630 -> [w649]
                  tunnel: w628 -> [w647] mode=indexing
                  n204 = call <instrlib>:"niScope Abort.vi"("instrument handle"=w647, "error in"=w649) -> ("instrument handle out"=w650:refnum<k15>, "error out"=w651:errorcluster)  [unwired: 12 in]
                  n205 = call <instrlib>:"niScope Close.vi"("instrument handle"=w650, "error in"=w651) -> ("error out"=w648:errorcluster)  [unwired: 13 in]
                }
                n206 = Empty String/Path?(string/path=w626) -> (empty?=w625:bool)
                n207 = case shown="False" w625 {
                  tunnel: w637 -> [w645 _]
                  tunnel: [w644 w646] -> w633
                  tunnel: w629 -> [w643 w646]
                  tunnel: w626 -> [w640 _]
                  frame False {
                    n208 = call <instrlib>:"niDCPower Abort With Channels.vi"("error in (no error)"=w643, "channel name"=w645, "instrument handle"=w640) -> ("error out"=w642:errorcluster, "instrument handle out"=w641:refnum<k15>)  [unwired: 7 in]
                    n209 = call <instrlib>:"niDCPower Close.vi"("error in (no error)"=w642, "instrument handle"=w641) -> ("error out"=w644:errorcluster)  [unwired: 9 in]
                  }
                  frame True {
                  }
                }
                n210 = call <instrlib>:"niDCPower Abort With Channels.vi"("error in (no error)"=w633, "channel name"=w634, "instrument handle"=w638) -> ("error out"=w636:errorcluster, "instrument handle out"=w635:refnum<k15>)  [unwired: 7 in]
                n211 = call <instrlib>:"niDCPower Close.vi"("error in (no error)"=w636, "instrument handle"=w635) -> ("error out"=w631:errorcluster)  [unwired: 9 in]
                n212 = Bundle By Name(cluster=w632, "Measurement Results.Status"="The measurement is performed successfully" ("message")) -> (w639:T3)
              }
              frame Error {
                # "Resets the device with default values whenever there is an error"
                n213 = Unbundle By Name(w668) -> ("Source out"=w663:refnum<k15>, "Source channel name"=w661:string, "Load out"=w660:refnum<k15>, "Load channel name"=w659:string, "Scopes out"=w656:refnum<k15>[])
                n214 = for {
                  shift-right: [w671] -> w657
                  shift-left: w658 -> [w672]
                  tunnel: w656 -> [w670] mode=indexing
                  n215 = call <instrlib>:"niScope Abort.vi"("instrument handle"=w670, "error in"=w672) -> ("instrument handle out"=w676:refnum<k15>, "error out"=w675:errorcluster)  [unwired: 12 in]
                  n216 = call <instrlib>:"niScope Reset.vi"("instrument handle"=w676, "error in"=w675) -> ("instrument handle out"=w674:refnum<k15>, "error out"=w673:errorcluster)  [unwired: 12 in]
                  n217 = call <instrlib>:"niScope Close.vi"("instrument handle"=w674, "error in"=w673) -> ("error out"=w671:errorcluster)  [unwired: 13 in]
                }
                n218 = call <instrlib>:"niDCPower Abort With Channels.vi"("error in (no error)"=w657, "channel name"=w659, "instrument handle"=w660) -> ("error out"=w653:errorcluster, "instrument handle out"=w652:refnum<k15>)  [unwired: 7 in]
                n219 = call <instrlib>:"niDCPower Reset With Channels.vi"("error in (no error)"=w653, "channel name"=w659, "instrument handle"=w652) -> ("error out"=w654:errorcluster, "instrument handle out"=w655:refnum<k15>)  [unwired: 7 in]
                n220 = call <instrlib>:"niDCPower Close.vi"("error in (no error)"=w654, "instrument handle"=w655) -> ("error out"=w662:errorcluster)  [unwired: 9 out]
                n221 = call <instrlib>:"niDCPower Abort With Channels.vi"("error in (no error)"=w662, "channel name"=w661, "instrument handle"=w663) -> ("error out"=w664:errorcluster, "instrument handle out"=w665:refnum<k15>)  [unwired: 7 in]
                n222 = call <instrlib>:"niDCPower Reset With Channels.vi"("error in (no error)"=w664, "channel name"=w661, "instrument handle"=w665) -> ("error out"=w667:errorcluster, "instrument handle out"=w666:refnum<k15>)  [unwired: 7 in]
                n223 = call <instrlib>:"niDCPower Close.vi"("error in (no error)"=w667, "instrument handle"=w666) -> ("error out"=w669:errorcluster)  [unwired: 9 out]
              }
            }
          }
        }
      }
    }
    frame "Power off the DUT" {
      # "Stops generation on the output channel and resets the channels to default values"
      n224 = Unbundle By Name(w706) -> ("Source resource name"=w708:string, "Load resource name"=w710:string)
      n225 = call <instrlib>:"niDCPower Initialize With Independent Channels.vi"("error in (no error)"=w716, "resource name"=w710) -> ("error out"=w692:errorcluster, "instrument handle out"=w691:refnum<k15>)  [unwired: 8 in]
      n226 = call-poly <instrlib>:"niDCPower Get Channel Name (Poly).vi"("error in (no error)"=w692, "index"="0", "instrument handle"=w691) -> ("error out"=w696:errorcluster, "name"=w693:string, "instrument handle out"=w694:refnum<k15>)  [unwired: 6 in]
      n227 = call <instrlib>:"niDCPower Configure Output Enabled.vi"("error in (no error)"=w696, "output enabled"=FALSE, "channel name"=w693, "instrument handle"=w694) -> ("error out"=w701:errorcluster, "instrument handle out"=w700:refnum<k15>)  [unwired: 6 in]
      n228 = call <instrlib>:"niDCPower Reset With Channels.vi"("error in (no error)"=w701, "channel name"=w693, "instrument handle"=w700) -> ("error out"=w697:errorcluster, "instrument handle out"=w698:refnum<k15>)  [unwired: 7 in]
      n229 = call <instrlib>:"niDCPower Close.vi"("error in (no error)"=w697, "instrument handle"=w698) -> ("error out"=w713:errorcluster)  [unwired: 9 out]
      n230 = call <instrlib>:"niDCPower Initialize With Independent Channels.vi"("error in (no error)"=w713, "resource name"=w708) -> ("error out"=w709:errorcluster, "instrument handle out"=w707:refnum<k15>)  [unwired: 8 in]
      n231 = call-poly <instrlib>:"niDCPower Get Channel Name (Poly).vi"("error in (no error)"=w709, "index"="0", "instrument handle"=w707) -> ("error out"=w712:errorcluster, "name"=w711:string, "instrument handle out"=w714:refnum<k15>)  [unwired: 6 in]
      n232 = call <instrlib>:"niDCPower Reset With Channels.vi"("error in (no error)"=w712, "channel name"=w711, "instrument handle"=w714) -> ("error out"=w719:errorcluster, "instrument handle out"=w718:refnum<k15>)  [unwired: 7 in]
      n233 = call <instrlib>:"niDCPower Close.vi"("error in (no error)"=w719, "instrument handle"=w718) -> ("error out"=w717:errorcluster)  [unwired: 9 out]
      n234 = Bundle By Name(cluster=w704, "Measurement Results.Status"="The DUT is powered OFF") -> (w703:T3)
    }
  }
  "error out" <- w4
  "measure call context out" <- w5
  n235 = Unbundle By Name(w2) -> ("Measurement Results"=→"measurement results":T1)
